vi "Create HTML.vi"(7 "FP Reference":refnum<class "Web Front Panel.lvclass">, 8 "error in (no error)":errorcluster, 10 "VI Identifier":string, 11 "Progress In":refnum<class "Progressbar.lvclass">) -> (0 "error out":errorcluster, 1 "js code for controls":string, 2 "js variables":string, 3 "Progress Out":refnum<class "Progressbar.lvclass">, 4 "script dependencies":string[](array[string]), 5 "HTML":string, 6 "js code for indicators":string)   [LabVIEW 2017, in "Front Panel Publisher.lvlib" / "Progressbar.lvclass"]
uses:
  Progressbar.lvclass
  Object_class/Object.lvclass
  Control_class/Control.lvclass
  Front Panel Publisher.lvlib
  Web Front Panel_class/Web Front Panel.lvclass
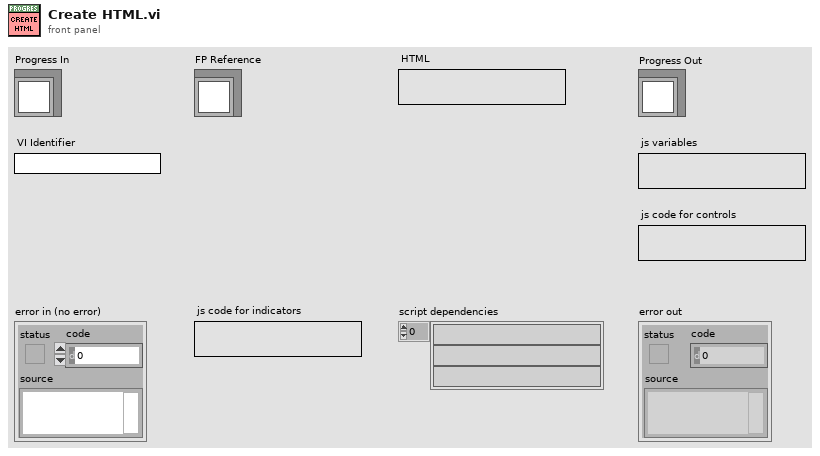
[diagram p1: front panel]
types:
  T1 = typedef "Front Panel Publisher.lvlib/Object.lvclass/Attributes.ctl" = cluster{"UID":i32, "Type":string, "Starting Location":T2, "Reference":refnum<vi>, "Cluster Component":bool, "Starting Rect Position":cluster{"Left":i16, "Top":i16}, "Owning Pane":refnum<vi>, "Master Total Rect Delta":T3}
  T2 = typedef "Front Panel Publisher.lvlib/Object.lvclass/Coordinates.ctl" = cluster{"Left":i32, "Top":i32, "Height":u32, "Width":u32}
  T3 = typedef "LVRectTypeDef.ctl" = cluster{"Left":i16, "Top":i16, "Right":i16, "Bottom":i16}
  T4 = typedef "Front Panel Publisher.lvlib/Control.lvclass/Attributes.ctl" = cluster{"Description":string, "Indicator":bool, "Default Value":variant, "Control Index":i32, "Label":refnum<class "Text.lvclass">, "Caption":refnum<class "Text.lvclass">, "Image b64":string, "No Control Index":bool, "Display Mode":T5}
  T5 = typedef "Front Panel Publisher.lvlib/Web Front Panel.lvclass/Enum - Control Display Mode.ctl" = enum16{"Value Only", "Value and Visibility", "Boolean Value Only", "Boolean Value and Visibility", "Control is Image", "Image and Visibility"}
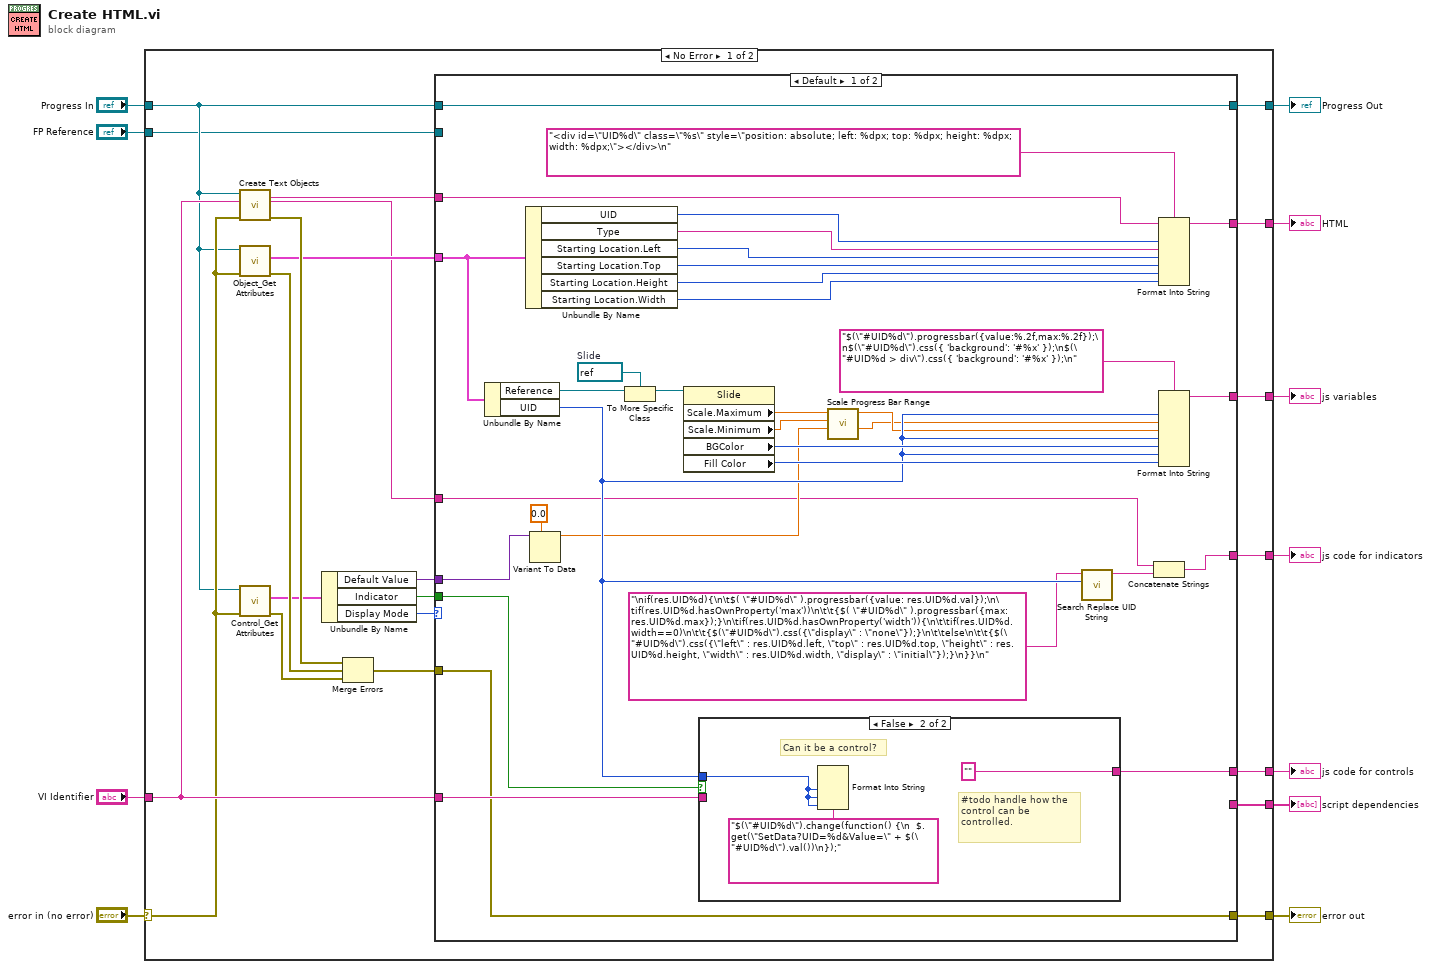
[diagram p0: block diagram]
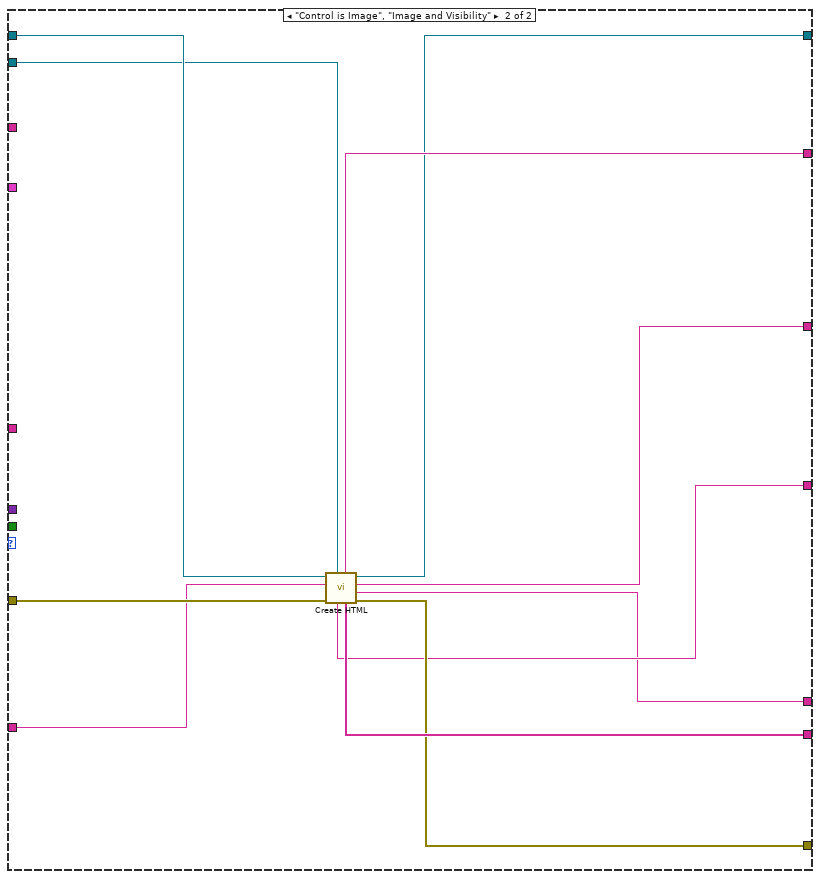
[diagram p3: hidden frame]
diagram:
  n1 = case shown="No Error" "error in (no error)" {
    selector: "error in (no error)" -> [w20 w83]
    tunnel: [w15 w83] -> w10
    tunnel: [w16 w82] -> w8
    tunnel: "Progress In" -> [w17 w82]
    tunnel: [w30 _] -> w7
    tunnel: [w26 _] -> w6
    tunnel: [w27 _] -> w5
    tunnel: "VI Identifier" -> [w24 _]
    tunnel: [w21 _] -> w3
    tunnel: [w14 _] -> w2
    tunnel: "FP Reference" -> [w12 _]
    frame No Error {
      n2 = call-dynamic "Create Text Objects.vi"("error in (no error)"=w20, "VI Name"=w24, "Control In"=w17) -> ("error out"=w31:errorcluster, "JS Indicator"=w13:string, "HTML"=w25:string)  [unwired: 5 in, 1 out]
      n3 = call "Object_Get Attributes.vi"("error in (no error)"=w20, "Object In"=w17) -> ("error out"=w32:errorcluster, "Object Attributes"=w22:T1)  [unwired: 7 in, 1 out]
      n4 = call "Control_Get Attributes.vi"("error in (no error)"=w20, "Control In"=w17) -> ("error out"=w33:errorcluster, "Control Attributes"=w29:T4)  [unwired: 7 in, 1 out]
      n5 = Unbundle By Name(w29) -> ("Default Value"=w23:variant, "Indicator"=w28:bool, "Display Mode"=w18:T5)
      n6 = Merge Errors(w31, w32, w33) -> (w19:errorcluster)
      n7 = case shown="Default" w18 {
        tunnel: [w62 w78] -> w30
        tunnel: w28 -> [w61 _]
        tunnel: [w60 w73] -> w27
        tunnel: [w36 w74] -> w26
        tunnel: w25 -> [w58 _]
        tunnel: w24 -> [w57 w80]
        tunnel: w23 -> [w56 _]
        tunnel: w22 -> [w49 _]
        tunnel: [w47 w72] -> w21
        tunnel: w19 -> [w37 w81]
        tunnel: w17 -> [w38 w79]
        tunnel: [w38 w77] -> w16
        tunnel: [w37 w75] -> w15
        tunnel: [_ w76] -> w14
        tunnel: w13 -> [w35 _]
        tunnel: w12 -> [_ w71]
        frame Default {
          w52 = refnum<vi> refnum  # Slide
          n8 = Unbundle By Name(w49) -> ("Reference"=w48:refnum<vi>, "UID"=w44:i32)
          n9 = Unbundle By Name(w49) -> ("UID"=w66:i32, "Type"=w65:string, "Starting Location.Left"=w64:i32, "Starting Location.Top"=w63:i32, "Starting Location.Height"=w54:u32, "Starting Location.Width"=w53:u32)
          n10 = Variant To Data(type=0.0, Variant=w56) -> (data=w40:dbl)  [unwired: 1 in, 1 out]
          n11 = To More Specific Class(target class=w52, reference=w48) -> (specific class reference=w51:refnum<vi>)  [unwired: 1 in, 1 out]
          n12 = property class="Slide"(reference=w51) -> ("Scale.Maximum"=w42:dbl, "Scale.Minimum"=w43:dbl, "BGColor"=w46:u32, "Fill Color"=w45:u32)  [unwired: 1 in, 2 out]
          n13 = case shown="False" w61 {
            tunnel: w44 -> [_ w69]
            tunnel: w57 -> [_ _]
            tunnel: [_ ""] -> w60
            frame True {
            }
            frame False {
              # "#todo handle how the control can be controlled."
              # "Can it be a control?"
              n14 = Format Into String(format string="$(\"#UID%d\").change(function() {\n  $.get(\"SetData?UID=%d&Value=\" + $(\"#UID%d\").val())\n});", w69, w69, w69) -> ()  [unwired: 2 in, 2 out]
            }
          }
          n15 = call "Scale Progress Bar Range.vi"("Value"=w40, "Minimum"=w43, "Maximum"=w42) -> ("Value Out"=w39:dbl, "Maximum Out"=w41:dbl)  [unwired: 7 in]
          n16 = call "Search Replace UID String.vi"("UID"=w44, "Input String"="\nif(res.UID%d){\n\t$( \"#UID%d\" ).progressbar({value: res.UID%d.val});\n\tif(res.UID%d.hasOwnProperty('max'))\n\t\t{$( \"#UID%d\" ).progressbar({max: res.UID%d.max});}\n\tif(res.UID%d.hasOwnProperty('width')){\n\t\tif(res.UID%d.width==0)\n\t\t{$(\"#UID%d\").css({\"display\" : \"none\"});}\n\t\telse\n\t\t{$(\"#UID%d\").css({\"left\" : res.UID%d.left, \"top\" : res.UID%d.top, \"height\" : res.UID%d.height, \"width\" : res.UID%d.width, \"display\" : \"initial\"});}\n}}\n") -> ("Output String"=w59:string)  [unwired: 9 in]
          n17 = Concatenate Strings(w35, w59) -> (w36:string)
          n18 = Format Into String(format string="<div id=\"UID%d\" class=\"%s\" style=\"position: absolute; left: %dpx; top: %dpx; height: %dpx; width: %dpx;\"></div>\n", initial string=w58, w66, w65, w64, w63, w54, w53) -> (resulting string=w62:string)  [unwired: 1 in, 1 out]
          n19 = Format Into String(format string="$(\"#UID%d\").progressbar({value:%.2f,max:%.2f});\n$(\"#UID%d\").css({ 'background': '#%x' });\n$(\"#UID%d > div\").css({ 'background': '#%x' });\n", w44, w39, w41, w44, w46, w44, w45) -> (resulting string=w47:string)  [unwired: 2 in, 1 out]
        }
        frame "Control is Image", "Image and Visibility" {
          n20 = call-parent "Create HTML.vi"("FP Reference"=w71, "error in (no error)"=w81, "VI Identifier"=w80, "Control In"=w79) -> ("error out"=w75:errorcluster, "js code for controls"=w73:string, "js variables"=w72:string, "Control Out"=w77:refnum<class "Progressbar.lvclass">, "script dependencies"=w76:string[], "HTML"=w78:string, "js code for indicators"=w74:string)  [unwired: 1 in]
        }
      }
    }
    frame Error {
    }
  }
  "error out" <- w10
  "Progress Out" <- w8
  "HTML" <- w7
  "js variables" <- w3
  "js code for controls" <- w5
  "script dependencies" <- w2
  "js code for indicators" <- w6
